vi "Test Main.vi"() -> ()   [LabVIEW 2015]
uses:
  State.ctl
  Data.ctl
panel:
  in  "texe":u32=10
  in  "twait":dbl=1.0
  in  "stop":bool
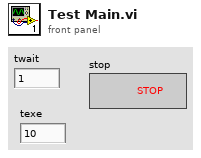
[diagram p1: front panel]
types:
  T1 = typedef "State.ctl" = enum16{"Configure", "Collect Data", "Wait", "Stop"}
  T2 = typedef "Data.ctl" = cluster{"Time":timestamp, "Voltage":dbl, "Amperage":dbl, "Wattage":dbl, "Power Factor":dbl, "Voltage Distortion":dbl, "Amperage Distortion":dbl, "Temperature":dbl}
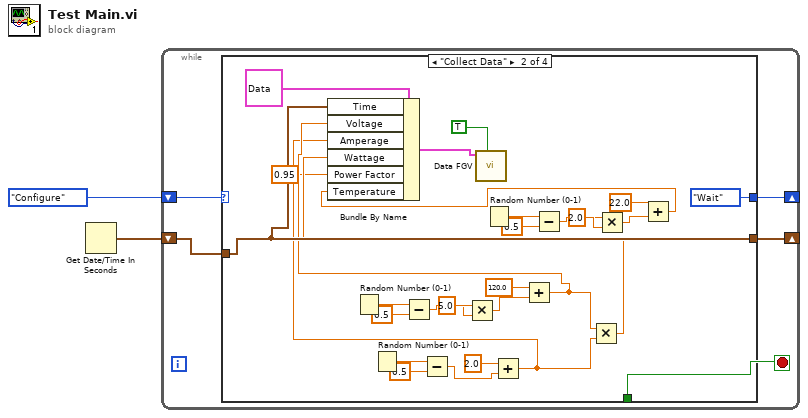
[diagram p0: block diagram]
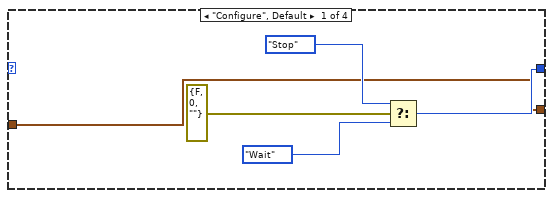
[diagram p2: hidden frame]
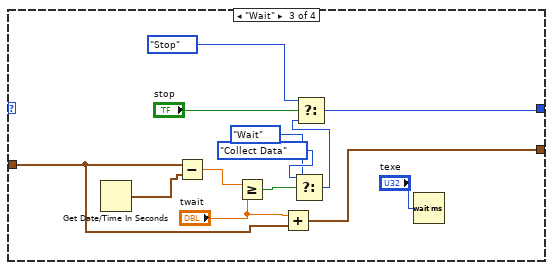
[diagram p3: hidden frame]
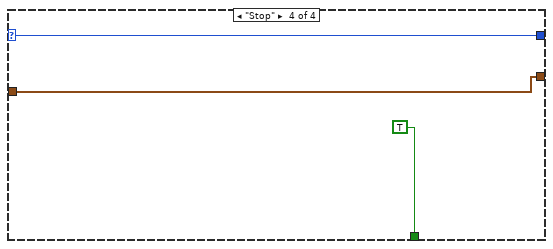
[diagram p4: hidden frame]
diagram:
  n1 = Get Date/Time In Seconds() -> (seconds since 1Jan1904=w2:timestamp)
  n2 = while {
    shift-right: [w3] -> _
    shift-left: w2 -> [w5]
    shift-right: [w6] -> _
    shift-left: State."Configure" -> [w7]
    stop <- w4 stop-if-true
    n3 = case shown="\"Collect Data\"" w7 {
      selector: w7 -> [_ _ _ w52]
      tunnel: [w9 State."Wait" w43 w52] -> w6
      tunnel: w5 -> [w8 w35 w42 w53]
      tunnel: [_ _ _ TRUE] -> w4
      tunnel: [w8 w35 w40 w53] -> w3
      frame "Configure", Default {
        n4 = Select(t=State."Stop", s=errorcluster {"status"=FALSE, "code"=0, "source"=""} ("error constant"), f=State."Wait") -> (s? t:f=w9:T1)
      }
      frame "Collect Data" {
        n5 = Random Number (0-1)() -> (number: 0 to 1=w34:dbl)
        n6 = Random Number (0-1)() -> (number: 0 to 1=w27:dbl)
        n7 = Subtract(x=w34, y=0.5) -> (x-y=w32:dbl)
        n8 = Subtract(x=w27, y=0.5) -> (x-y=w25:dbl)
        n9 = Multiply(x=w32, y=5.0 ("x")) -> (x*y=w30:dbl)
        n10 = Random Number (0-1)() -> (number: 0 to 1=w17:dbl)
        n11 = Add(x=2.0, y=w25) -> (x+y=w22:dbl)
        n12 = Add(x=120.0, y=w30) -> (x+y=w23:dbl)
        n13 = Subtract(x=w17, y=0.5) -> (x-y=w19:dbl)
        n14 = Multiply(x=w23, y=w22) -> (x*y=w24:dbl)
        n15 = Multiply(x=w19, y=2.0 ("x")) -> (x*y=w16:dbl)
        n16 = Add(x=22.0, y=w16) -> (x+y=w14:dbl)
        n17 = Bundle By Name(cluster=T2 {"Time"=timestamp(0 s since 1904-01-01), "Voltage"=0.0, "Amperage"=0.0, "Wattage"=0.0, "Power Factor"=0.0, "Voltage Distortion"=0.0, "Amperage Distortion"=0.0, "Temperature"=0.0} ("Data In"), "Time"=w35, "Voltage"=w23, "Amperage"=w22, "Wattage"=w24, "Power Factor"=0.95, "Temperature"=w14) -> (w13:T2)
        n18 = call "Data FGV.vi"("Write?"=TRUE, "Data In"=w13) -> ()  [unwired: 9 in, 1 out]
      }
      frame "Wait" {
        n19 = Get Date/Time In Seconds() -> (seconds since 1Jan1904=w48:timestamp)
        n20 = Subtract(x=w42, y=w48) -> (x-y=w47:dbl)
        n21 = Greater Or Equal?(x=w47, y="twait") -> (x >= y?=w46:bool)
        n22 = Add(x="twait", y=w42) -> (x+y=w40:timestamp)
        n23 = Select(t=State."Collect Data", s=w46, f=State."Wait") -> (s? t:f=w44:T1)
        n24 = Select(t=State."Stop", s="stop", f=w44) -> (s? t:f=w43:T1)
        n25 = Wait (ms)(milliseconds to wait="texe") -> ()  [unwired: 1 out]
      }
      frame "Stop" {
      }
    }
  }
